vi "Timed Messaging Test Core.vi"(4 "expected":i32=5, 6 "notification":T1=enum."Send next copy now and stop all further copies", 8 "error in":errorcluster, 11 "Test Case In":refnum<class "Messaging Tests.lvclass">) -> (0 "error out":errorcluster, 3 "Test Case Out":refnum<class "Messaging Tests.lvclass">)   [LabVIEW 2020, in "Messaging Tests.lvlib" / "Messaging Tests.lvclass"]
uses:
  Messaging Tests.lvclass
  Core/ActorFramework/Time-Delayed Send Message/Time-Delay Override Options.ctl
  C:/Program Files/National Instruments/LabVIEW 2024/vi.lib/Astemes/LUnit/Test Case.lvclass
  TestActor/Increment Msg/Increment Msg.lvclass/Increment Msg.ctl
  Core/ActorFramework/Message Queue/Message Queue.lvclass/Message Queue.ctl
  Core/ActorFramework/Message Dequeuer/Message Dequeuer.lvclass/Message Dequeuer.ctl
  <vilib>/Astemes/LUnit/Test Case.lvclass/Test Case.ctl
  9e91c561-e7f8-4100-8a99-98b4b15ba9ac.vi
  8f729260-0eef-4fe8-8e95-6fe6bb364e16.vi
  b6e3af16-1b80-47bf-845f-a97468ea47c9.vi
  <vilib>/Astemes/LUnit/Append Pass Result.vi
  <vilib>/Astemes/LUnit/Append Fail Result.vi
  b6e3af16-1b80-47bf-845f-a97468ea47c9.vi/9c5d11cd-9439-4240-a1ee-d9baace9c924.vi
  <vilib>/Astemes/LUnit/Run In UI.vi
  <vilib>/Utility/error.llb/Clear Errors.vi
  TestActor/Increment Msg/Increment Msg.lvclass
  C:/Users/J63553/Projects/_LabVIEW Community/actor-framework/Core/ActorFramework/Message/Message.lvclass
  Core/ActorFramework/Message Priority Queue/Priority Dequeue.vi
  Core/ActorFramework/Message Queue/Message Queue.lvclass
  Core/ActorFramework/Message Dequeuer/Message Dequeuer.lvclass
  Core/ActorFramework/Actor Framework.lvlib
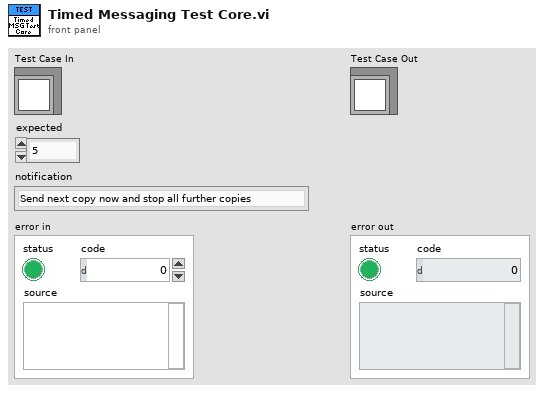
[diagram p1: front panel]
types:
  T1 = typedef "Actor Framework.lvlib/Time-Delay Override Options.ctl" = enum16{"Send next copy now", "Skip next scheduled copy", "Send next copy now and stop all further copies", "Stop all further copies"}
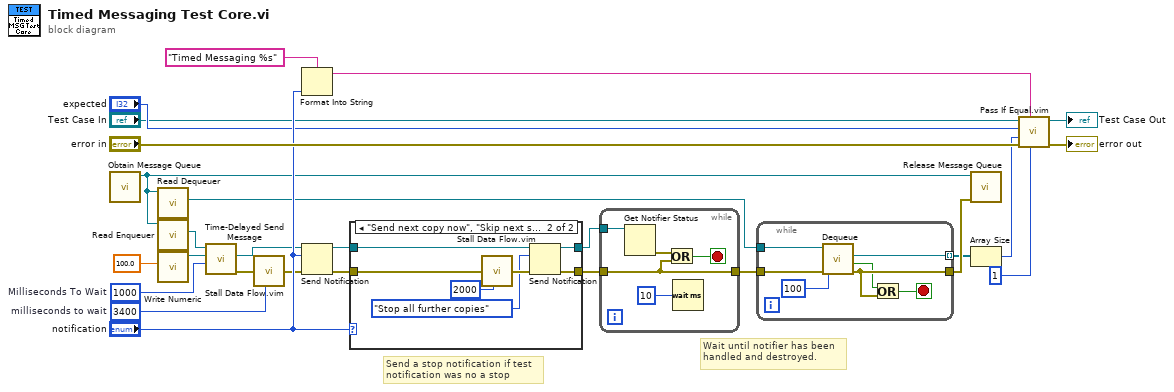
[diagram p0: block diagram]
diagram:
  w10 = u32 3400  # milliseconds to wait
  w16 = 1000  # Milliseconds To Wait
  # "Send a stop notification if test\nnotification was no a stop"
  # "Wait until notifier has been\nhandled and destroyed."
  n1 = call "Obtain Message Queue.vi"() -> ("Message Queue"=w11:refnum<class "Message Queue.lvclass">)  [unwired: 10 in, 1 out]
  n2 = call "Read Dequeuer.vi"("Message Queue"=w11) -> ("Message Dequeuer"=w12:refnum<class "Message Dequeuer.lvclass">)  [unwired: 10 in]
  n3 = call "Read Enqueuer.vi"("Message Queue"=w11) -> ("Message Enqueuer"=w13:refnum<class "Message Enqueuer.lvclass">)  [unwired: 10 in]
  n4 = call "Write Numeric.vi"("Numeric"=100.0) -> ("Increment Msg out"=w17:refnum<class "Increment Msg.lvclass">)  [unwired: 10 in]
  n5 = call "Time-Delayed Send Message.vi"("Milliseconds To Wait"=w16, "Message"=w17, "Message Enqueuer"=w13) -> ("error out"=w25:errorcluster, "Delivery Notifier"=w15:refnum<notifier>)  [unwired: 7 in]
  n6 = call "Stall Data Flow.vim"("value in"=w25, "milliseconds to wait"=w10) -> ("value out"=w22:errorcluster)  [unwired: 1 out]
  n7 = Format Into String(format string="Timed Messaging %s", "notification") -> (resulting string=w2:string)  [unwired: 2 in, 1 out]
  n8 = Send Notification(notification="notification", notifier=w15, error in (no error)=w22) -> (notifier out=w6:refnum<notifier>, error out=w20:errorcluster)
  n9 = case shown="\"Send next copy now\", \"Skip next scheduled copy\"" "notification" {
    tunnel: w20 -> [w29 w35]
    tunnel: w6 -> [w28 w31]
    tunnel: [w29 w34] -> w19
    tunnel: [w28 w30] -> w5
    frame "Send next copy now and stop all further copies", "Stop all further copies" {
    }
    frame "Send next copy now", "Skip next scheduled copy" {
      n10 = call "Stall Data Flow.vim"("value in"=w35, "milliseconds to wait"=u32 2000) -> ("value out"=w36:errorcluster)  [unwired: 1 out]
      n11 = Send Notification(notification=Time-Delay_Override_Options."Stop all further copies", notifier=w31, error in (no error)=w36) -> (notifier out=w30:refnum<notifier>, error out=w34:errorcluster)
    }
  }
  n12 = while {
    tunnel: w5 -> [w39]
    tunnel: [w40] -> w24
    tunnel: w19 -> [w40]
    stop <- w37 stop-if-true
    n13 = Get Notifier Status(notifier=w39) -> (error out=w41:errorcluster)  [unwired: 1 in, 4 out]
    n14 = Or(x=w41, y=w40) -> (x .or. y?=w37:bool)
    n15 = Wait (ms)(milliseconds to wait=u32 10) -> ()  [unwired: 1 out]
  }
  n16 = while {
    tunnel: w12 -> [w46]
    tunnel: w24 -> [w48]
    tunnel: [w44] -> w14 mode=indexing
    tunnel: [w47] -> w23
    stop <- w42 stop-if-true
    n17 = call "Dequeue.vi"("error in (no error)"=w48, "timeout in ms (-1)"=100, "Message Dequeuer in"=w46) -> ("error out"=w47:errorcluster, "timed out?"=w43:bool, "Message"=w44:refnum<class "Message.lvclass">)  [unwired: 4 in, 2 out]
    n18 = Or(x=w43, y=w47) -> (x .or. y?=w42:bool)
  }
  n19 = call "Release Message Queue.vi"("error in (no error)"=w23, "Message Queue"=w11) -> ()  [unwired: 8 in, 2 out]
  n20 = Array Size(array=w14) -> (size(s)=w9:i32)
  n21 = call "Pass If Equal.vim"("Delta"=1, "Description"=w2, "error in (no error)"="error in", "Actual"=w9, "Expected"="expected", "LUnit Test Case In"="Test Case In") -> ("error out"=→"error out":errorcluster, "LUnit Test Case Out"=→"Test Case Out":refnum<class "Messaging Tests.lvclass">)  [unwired: 4 in]
